vi "cw_1_9.vi"() -> ()   [LabVIEW 2022 SP3]
panel:
  out "Number in Range":bool
  in  "Temp":dbl(slide) scale=0.0..1000.0
  in  "Lower Limit":dbl(knob) scale=0.0..1000.0
  in  "Upper Limit":dbl(knob) scale=0.0..1000.0
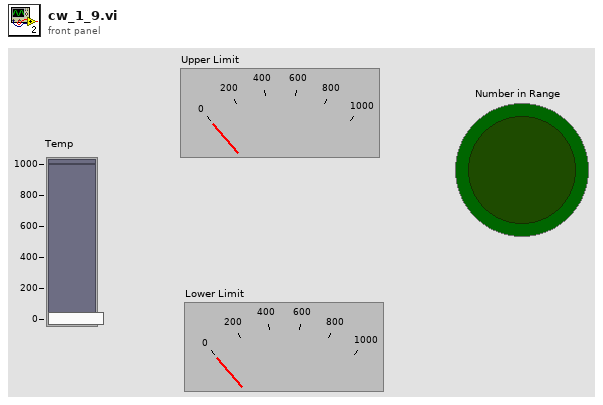
[diagram p1: front panel]
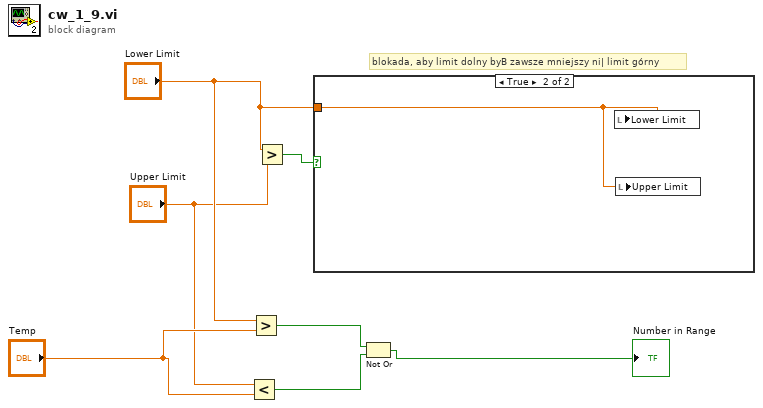
[diagram p0: block diagram]
diagram:
  # "blokada, aby limit dolny byB zawsze mniejszy ni| limit górny"
  n1 = Less?(x="Upper Limit", y="Temp") -> (x < y?=w4:bool)
  n2 = Greater?(x="Lower Limit", y="Temp") -> (0:w5:bool)
  n3 = Greater?(x="Lower Limit", y="Upper Limit") -> (0:w7:bool)
  n4 = case shown="True" w7 {
    tunnel: "Lower Limit" -> [_ w8]
    frame False {
    }
    frame True {
      n5 = local write "Lower Limit"(w8) -> ()
      n6 = local write "Upper Limit"(w8) -> ()
    }
  }
  n7 = Not Or(1:w4, 2:w5) -> (0:→"Number in Range":bool)
